vi "Wash Display - Step to Indicator.vi"(8 "error in (no error)":errorcluster, 11 "Wash Step":T2) -> (0 "error out":errorcluster, 3 "Wash Steps":T1)   [LabVIEW 2017]
doc: "SubVI for translate Wash Step to Wash Indicators.\n[Covers: SS5]"
uses:
  Controller/Controls/Controller - Wash Step.ctl
  Entry Console View/Controls/Entry Console - Wash Steps.ctl
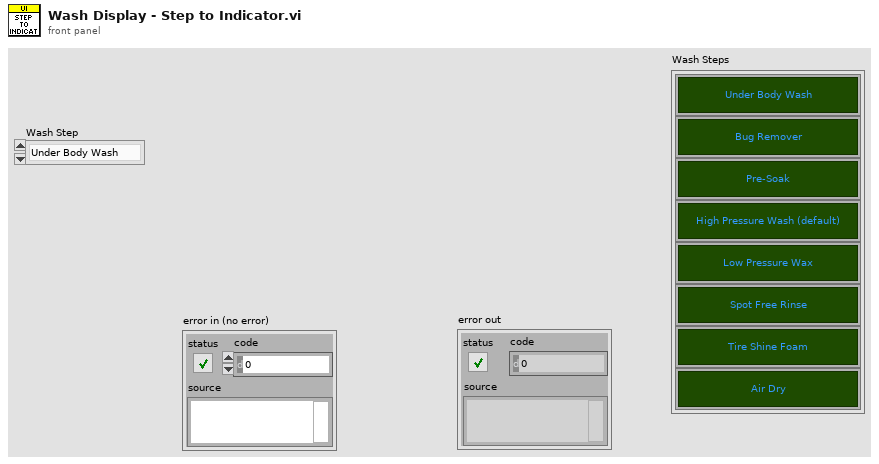
[diagram p1: front panel]
types:
  T1 = typedef "Entry Console - Wash Steps.ctl" = cluster{"Under Body Wash":bool, "Bug Remover":bool, "Pre-Soak":bool, "High Pressure Wash":bool, "Low Pressure Wax":bool, "Spot Free Rinse":bool, "Tire Shine Foam":bool, "Air Dry":bool}
  T2 = typedef "Controller - Wash Step.ctl" = enum16{"Under Body Wash", "Bug Remover", "Pre-Soak", "High Pressure Wash", "Low Pressure Wax", "Spot Free Rinse", "Tire Shine Foam", "Air Dry"}
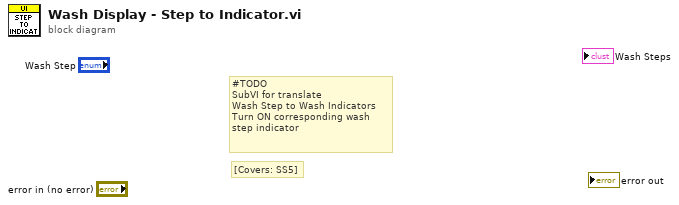
[diagram p0: block diagram]
diagram:
  # "[Covers: SS5]"
  # "#TODO\nSubVI for translate\nWash Step to Wash Indicators\nTurn ON corresponding wash \nstep indicator"
